vi "get cause.vi"(11 "exception in":T1 {"code" format="%.0x"}) -> (2 "cause":T1 {"code" format="%.0x"}, 3 "exception out":T1 {"code" format="%.0x"})   [LabVIEW 2013, in "exception.lvlib"]
uses:
  exception.lvlib
  exception.ctl
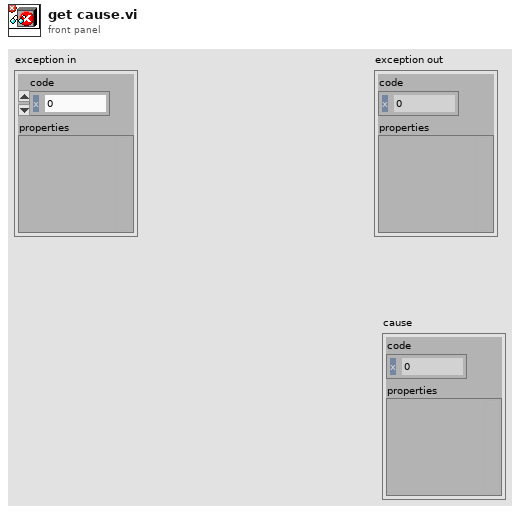
[diagram p1: front panel]
types:
  T1 = typedef "exception.lvlib/exception.ctl" = cluster{"code":i32, "properties":variant}
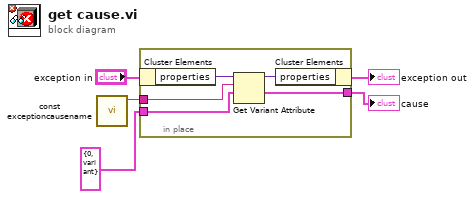
[diagram p0: block diagram]
diagram:
  n1 = call "const exceptioncausename.vi"() -> ("label"=w2:string)  [unwired: 11 in]
  n2 = in-place {
    in-place-border: w2 -> [w8]
    in-place-border: T1 {"code"=0, "properties"=variant} ("cause") -> [w7]
    in-place-border: [w6] -> w1
    n3 = in-place-cluster #1("exception in") -> ("properties"=w10:variant)
    n4 = Get Variant Attribute(Variant=w10, name=w8, default value (empty Variant)=w7) -> (duplicate Variant=w9:variant, value=w6:T1)  [unwired: 1 in, 2 out]
    n5 = in-place-cluster #1("properties"=w9) -> (→"exception out":T1)
  }
  "cause" <- w1
